vi "OscilloscopeRead.vi"(8 "error in (no error)":errorcluster, 9 "channelsOsc":i16[](array[numeric])=[1, 2] min=0 max=3 step=1, 10 "ON/OFF":bool=TRUE, 11 "Control-Client in":refnum<class "Control-Client.lvclass">) -> (0 "error out":errorcluster, 3 "Control-Client out":refnum<class "Control-Client.lvclass">)   [LabVIEW 2015, in "Control-Client.lvclass"]
uses:
  Control-Client.lvclass
  dependecies/ControlsVIs/Clusters-def/Message types.ctl
  dependecies/ControlsVIs/Clusters-def/OSc-Demand-Read.ctl
  Oscilloscope/Oscilloscope.lvclass
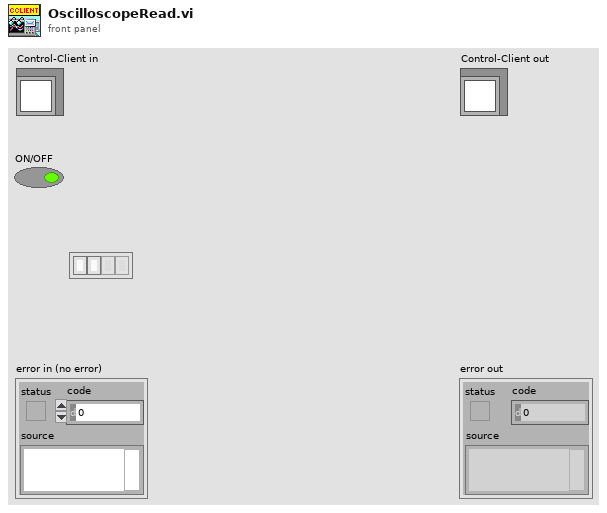
[diagram p1: front panel]
types:
  T1 = typedef "Oscilloscope.lvclass/OSc-Demand-Read.ctl" = cluster{"ON/OFF":bool, "Channels":u16[]}
  T2 = typedef "Message types.ctl" = string
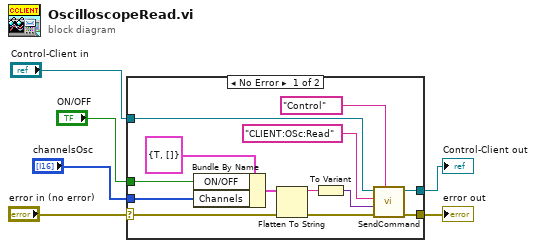
[diagram p0: block diagram]
diagram:
  n1 = case shown="No Error" "error in (no error)" {
    selector: "error in (no error)" -> [w13 w21]
    tunnel: [w12 w21] -> w5
    tunnel: [w11 w20] -> w3
    tunnel: "Control-Client in" -> [w19 w20]
    tunnel: "ON/OFF" -> [w9 _]
    tunnel: "channelsOsc" -> [w7 _]
    frame No Error {
      n2 = Bundle By Name(cluster=T1 {"ON/OFF"=TRUE, "Channels"=[]}, "ON/OFF"=w9, "Channels"=w7) -> (w8:T1)
      n3 = Flatten To String(anything=w8, error in (no error)=w13) -> (data string=w15:string, error out=w16:errorcluster)  [unwired: 2 in, 1 out]
      n4 = To Variant(anything=w15) -> (Variant=w18:variant)
      n5 = call "SendCommand.vi"("Message type"=T2 "Control", "error in (no error)"=w16, "data"=w18, "Command"="CLIENT:OSc:Read" ("chaîne"), "Control-Client in"=w19) -> ("error out"=w12:errorcluster, "Control-Client out"=w11:refnum<class "Control-Client.lvclass">)  [unwired: 5 in]
    }
    frame Error {
    }
  }
  "error out" <- w5
  "Control-Client out" <- w3
